vi "GenerateFilenames.vi"(8 "file number":i32, 10 "filename":string, 11 "Path":path) -> (3 "Filepath":path)   [LabVIEW 2019]
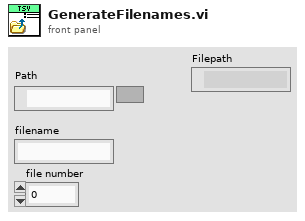
[diagram p1: front panel]
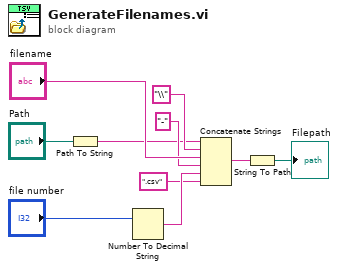
[diagram p0: block diagram]
diagram:
  n1 = Path To String(path="Path") -> (string=w1:string)
  n2 = Number To Decimal String(number="file number") -> (decimal integer string=w6:string)  [unwired: 1 in]
  n3 = Concatenate Strings(w1, "\\" ("string"), "filename", "-" ("string"), w6, ".csv" ("string")) -> (w3:string)
  n4 = String To Path(string=w3) -> (path=→"Filepath":path)
